vi "6517b+lakeshore335.vi"(8 "Set Temp Point":dbl=10.0, 11 "335 VISA resource name":refnum<visa-resource-name>="GPIB0::12::INSTR") -> ()   [LabVIEW 2019]
uses:
  lib/Lake Shore 335/Lake Shore 335.lvlib
  SubVI/SubVI.lvlib
  lib/Keithley 6517/Keithley 6517.lvlib
  <vilib>/Utility/file.llb/Write To Spreadsheet File (DBL).vi
  <vilib>/Utility/file.llb/Read From Spreadsheet File (DBL).vi
panel:
  out "Measurement":T1 {"Measurement" format="%.6e"}
  in  "VISA resource name":refnum<visa-resource-name>
  in  "采集最小间隔（ms）":u32
  in  "6157B":bool=TRUE
  out "Graph 2":cluster{"Y":dbl[], "Y":dbl[]}[](graph)
  out "Graph 1":cluster{"Y":dbl[], "Y":dbl[]}[](graph)
  in  "Y":u16(ring)=1 items=["时间", "通道A", "通道B", "电压", "电流", "电阻"]
  in  "X 2":u16(ring) items=["时间", "通道A", "通道B", "电压", "电流", "电阻"]
  in  "Y 2":u16(ring)=2 items=["时间", "通道A", "通道B", "电压", "电流", "电阻"]
  in  "X":u16(ring) items=["时间", "通道A", "通道B", "电压", "电流", "电阻"]
  out "Graph 3":cluster{"Y":dbl[], "Y":dbl[]}[](graph)
  out "Graph 4":cluster{"Y":dbl[], "Y":dbl[]}[](graph)
  in  "Y 3":u16(ring)=1 items=["时间", "通道A", "通道B", "电压", "电流", "电阻"]
  in  "X 3":u16(ring) items=["时间", "通道A", "通道B", "电压", "电流", "电阻"]
  in  "X 4":u16(ring) items=["时间", "通道A", "通道B", "电压", "电流", "电阻"]
  in  "Y 4":u16(ring)=2 items=["时间", "通道A", "通道B", "电压", "电流", "电阻"]
  in  "STOP":bool=TRUE
  out "date/time string":string="20171114204549"
  in  "file path (dialog if empty)":path
  in  "Range (0:Off)":u16(ring) items=["Off", "Low (On)", "Medium", "High"]
  in  "Heater Output (1:1)":u16(ring)=1 items=["1"=1, "2"=2]
  in  "Mode (0:Off)":u16(ring)=1 items=["Off", "Closed Loop PID", "Zone", "Open Loop", "Monitor Out", "Warmup Supply"]
  in  "Output Type (0:Current)":u16(ring) items=["Current", "Voltage"]
  in  "Power Up Enable (F: Off)":bool=TRUE
  in  "Input (0:None)":u16(ring)=2 items=["None", "A", "B"]
  in  "Max Current (0:User Specified)":u16(ring)=4 items=["User Specified", "0.707 A", "1.0 A", "1.141 A", "1.732 A"]
  in  "Max User Current (1.732)":dbl=1.0 format="%.3f"
  out "Heater Range":u16(ring) items=["Off", "Low (On)", "Medium", "High"]
  out "Heater Status":u16(ring) items=["No Error", "Heater Open Load", "Heater Short"]
  in  "Ramp Rate (0.0)":dbl=3.0 format="%.1f"
  in  "Enable Setpoint \nRamping (F: Off)":bool=TRUE
  # "K"
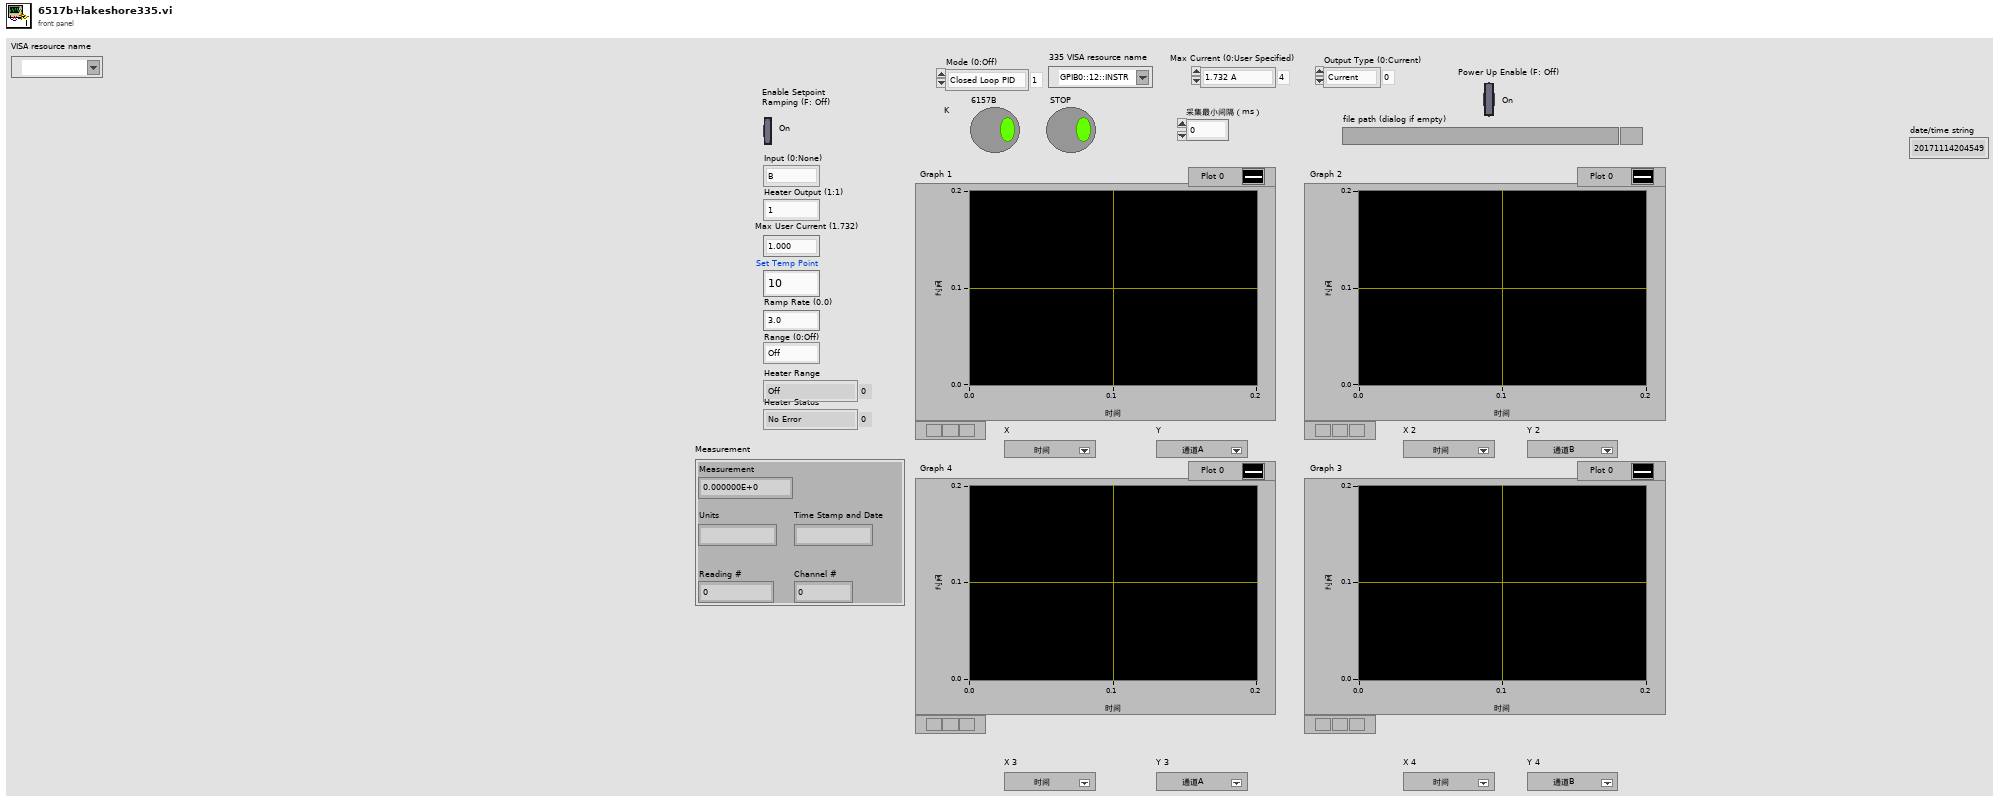
[diagram p1: front panel]
types:
  T1 = cluster{"Measurement":dbl, "Units":string, "Time Stamp and Date":string, "Reading #":dbl, "Channel #":dbl}
  T2 = enum16{"open", "replace", "create", "open or create", "replace or create", "replace or create with confirmation"}
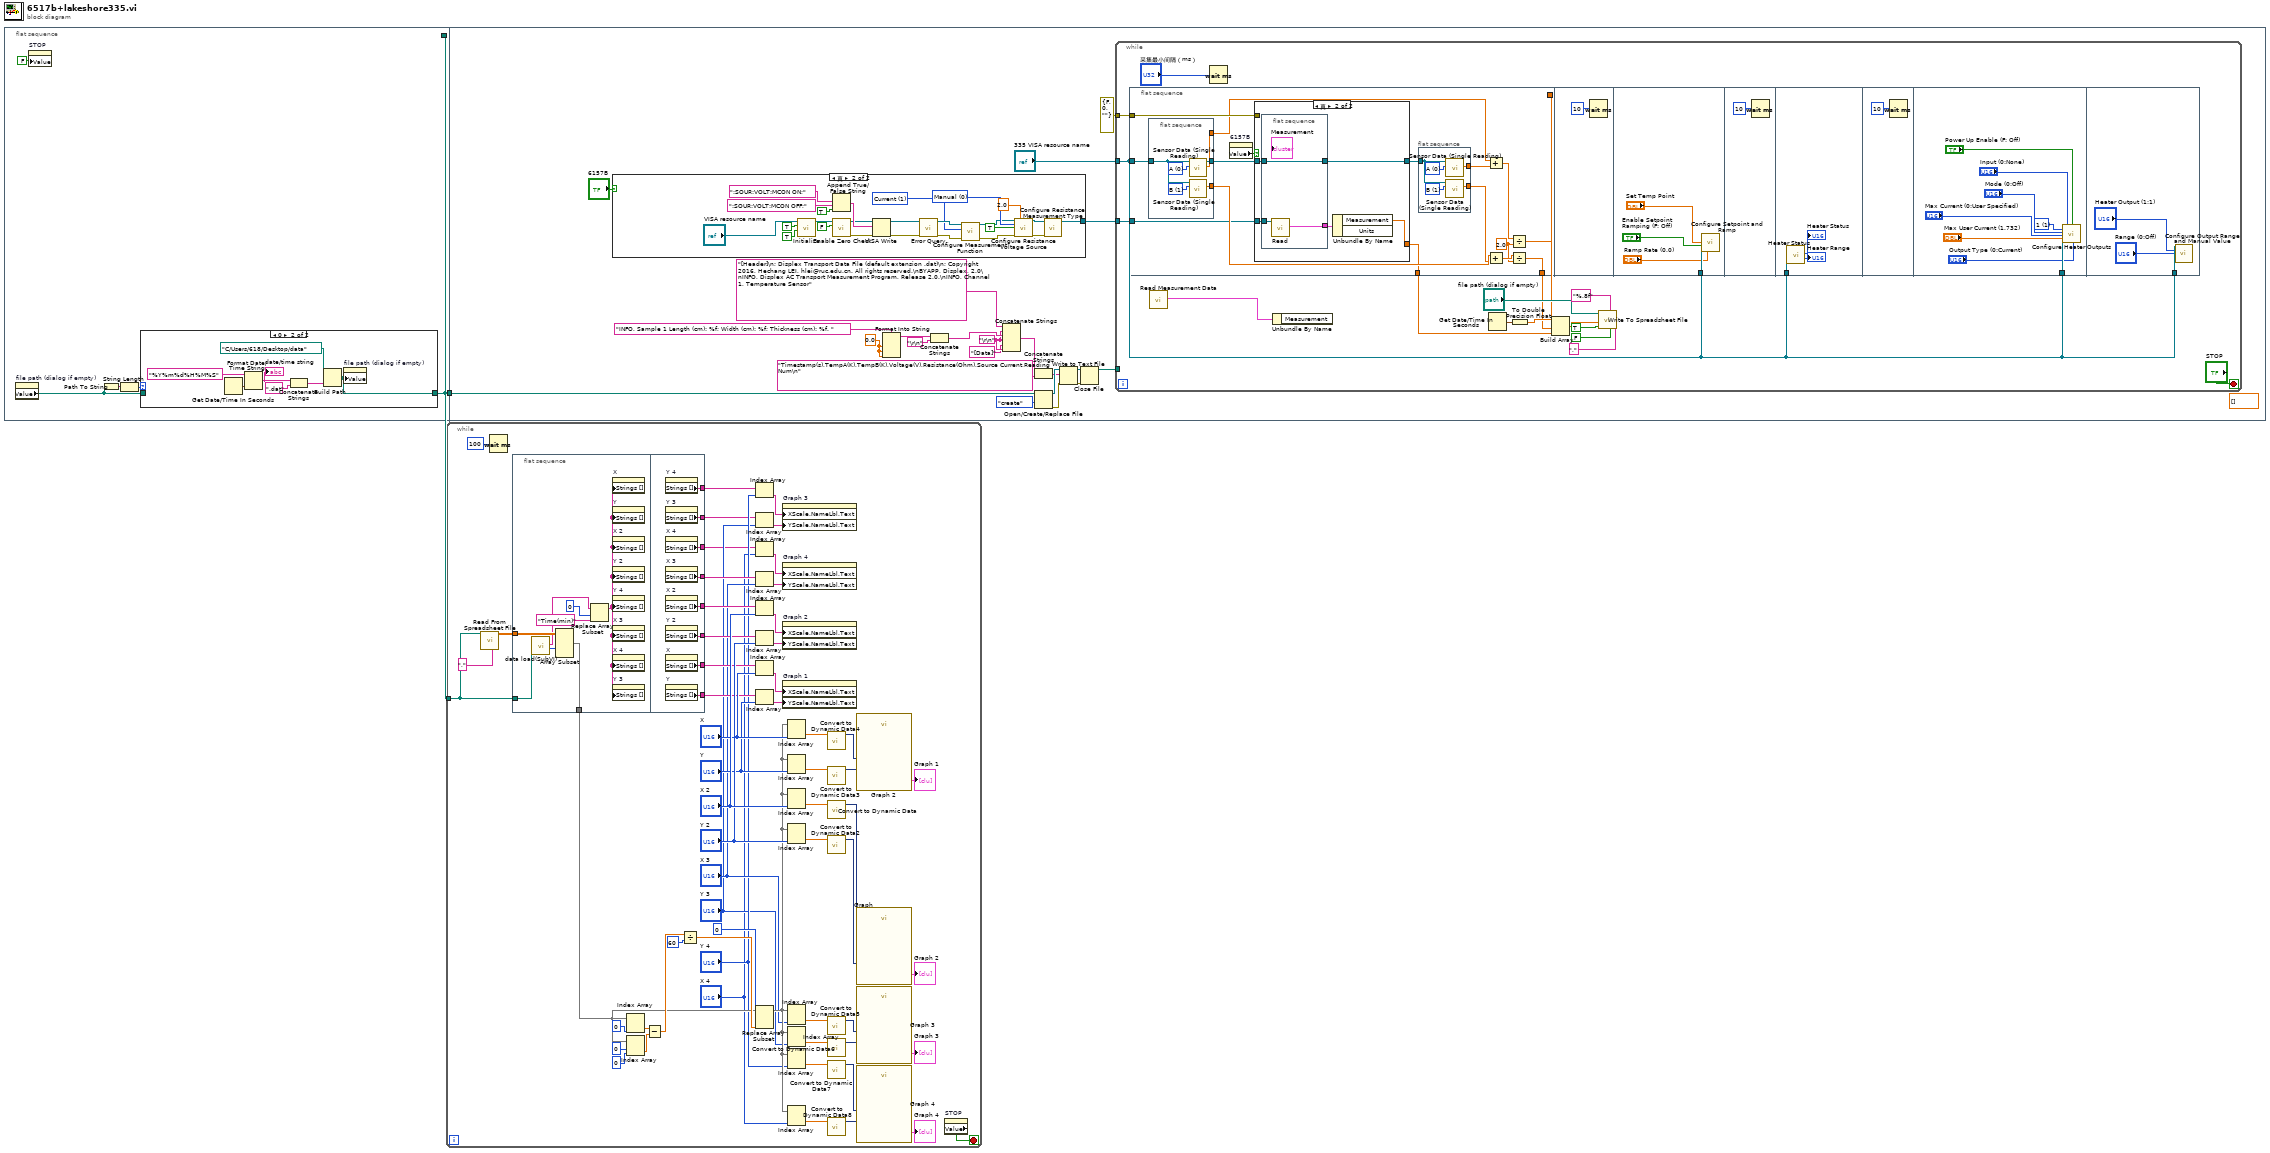
[diagram p0: block diagram]
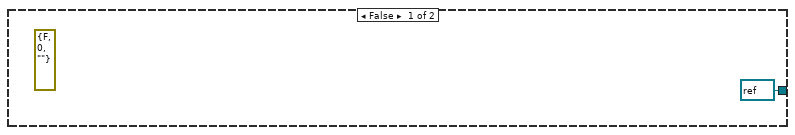
[diagram p3: hidden frame]
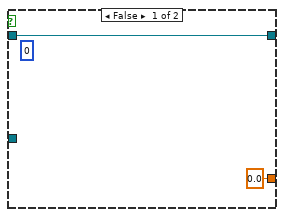
[diagram p4: hidden frame]
diagram:
  n1 = flat-sequence {
    tunnel: [w3] -> w1
    tunnel: [w3] -> w2
    tunnel: w2 -> [w35]
    frame #0 {
      n2 = property on="file path (dialog if empty)" class="Path"() -> ("Value"=w4:path)  [unwired: 2 in, 2 out]
      n3 = property on="STOP" class="Bool (严格)"("Value"=FALSE ("Boolean")) -> ()  [unwired: 2 in, 2 out]
      n4 = Path To String(path=w4) -> (string=w7:string)
      n5 = String Length(string=w7) -> (length=w6:i32)
      n6 = case shown="0" w6 {
        tunnel: [w8 w9] -> w3
        tunnel: w4 -> [w8 _]
        frame 1, Default {
        }
        frame 0 {
          n7 = Get Date/Time In Seconds() -> (seconds since 1Jan1904=w15:timestamp)
          n8 = Format Date/Time String(time format string (%c)="%Y%m%d%H%M%S", seconds (now)=w15) -> (date/time string=w10:string)  [unwired: 1 in]
          "date/time string" <- w10
          n9 = Concatenate Strings(w10, ".dat" ("string")) -> (w11:string)
          n10 = Build Path(base path=path "C:/Users/618/Desktop/data" ("文件夹路径"), name or relative path=w11) -> (appended path=w9:path)
          n11 = property on="file path (dialog if empty)" class="Path"("Value"=w9) -> ()  [unwired: 2 in, 2 out]
        }
      }
    }
    frame #1 {
      w24 = 0.0 ("输入 1")
      w27 = "\r\n"
      (unwired) dbl[] []
      n12 = case shown="真" "6157B" {
        tunnel: [refnum<visa-resource-name> refnum ("VISA resource name out") w39] -> w17
        frame False {
          (unwired) errorcluster {"status"=FALSE, "code"=0, "source"=""} ("error out")
        }
        frame True {
          w44 = 1 items=["Voltage", "Current", "Resistance", "Charge"] ("Measurement Function (0: Voltage)")
          w50 = 0 items=["Manual", "Auto"] ("Voltage Source Mode (0: Manual)")
          n13 = call "Initialize.vi"("Reset (True)"=TRUE, "ID Query (True)"=TRUE, "VISA resource name"="VISA resource name") -> ("VISA resource name out"=w42:refnum<visa-resource-name>)  [unwired: 7 in, 1 out]
          n14 = Append True/False String(1:TRUE ("Enable LO Connection (F: Disable)"), 2:":SOUR:VOLT:MCON OFF;", 3:":SOUR:VOLT:MCON ON;") -> (0:w59:string)  [unwired: 1 in]
          n15 = call "Enable Zero Check.vi"("Enable Zero Check (T: Enable)"=FALSE, "VISA resource name"=w42) -> ("error out"=w57:errorcluster, "VISA resource name out"=w58:refnum<visa-resource-name>)  [unwired: 8 in]
          n16 = VISA Write(VISA resource name=w58, write buffer=w59, error in (no error)=w57) -> (VISA resource name out=w56:refnum<visa-resource-name>, error out=w55:errorcluster)  [unwired: 1 out]
          n17 = call "Error Query.vi"("error in (no error)"=w55, "VISA resource name"=w56) -> ("error out"=w48:errorcluster, "VISA resource name out"=w47:refnum<visa-resource-name>)  [unwired: 6 in, 2 out]
          n18 = call "Configure Measurement Function.vi"("error in (no error)"=w48, "Measurement Function (0: Voltage)"=w44, "VISA resource name"=w47) -> ("error out"=w45:errorcluster, "VISA resource name out"=w46:refnum<visa-resource-name>)  [unwired: 7 in]
          n19 = call "Configure Resistance Voltage Source.vi"("VISA resource name"=w46, "Voltage Source Level (0.000000E+0)"=2.0, "Voltage Source Mode (0: Manual)"=w50, "Enable Voltage Source (F: Disable)"=TRUE, "error in (no error)"=w45) -> ("VISA resource name out"=w53:refnum<visa-resource-name>, "error out"=w52:errorcluster)  [unwired: 9 in]
          n20 = call "Configure Resistance Measurement Type.vi"("error in (no error)"=w52, "VISA resource name"=w53) -> ("VISA resource name out"=w39:refnum<visa-resource-name>)  [unwired: 8 in, 1 out]
        }
      }
      n21 = Format Into String(format string="INFO, Sample 1 Length (cm): %f; Width (cm): %f; Thickness (cm): %f. " ("string"), w24, w24, w24) -> (resulting string=w31:string)  [unwired: 2 in, 1 out]
      n22 = Concatenate Strings(w31, "\r\n") -> (w32:string)
      n23 = Concatenate Strings("[Header]\n; Displex Transport Data File (default extension .dat)\n; Copyright 2016, Hechang LEI, hlei@ruc.edu.cn. All rights reserved.\nBYAPP, Displex, 2.0\nINFO, Displex AC Transport Measurement Program, Release 2.0.\nINFO, Channel 1, Temperature Sensor" ("string"), w27, w32, w27, "[Data]" ("string"), w27) -> (w33:string)
      n24 = Concatenate Strings(w33, "Timestamp(s),TempA(K),TempB(K),Voltage(V),Resistance(Ohm),Source Current,Reading Num\n" ("字符串")) -> (w23:string)
      n25 = Open/Create/Replace File(file path (use dialog)=w35, operation (0:open)=T2."create") -> (refnum out=w34:refnum<file>, error out=w20:errorcluster)  [unwired: 4 in, 1 out]
      n26 = Write to Text File(file (use dialog)=w34, text=w23, error in=w20) -> (refnum out=w22:refnum<file>, error out=w21:errorcluster)  [unwired: 1 in, 1 out]
      n27 = Close File(refnum=w22, error in=w21) -> (path=w19:path)  [unwired: 1 out]
      n28 = while {
        tunnel: "335 VISA resource name" -> [w79]
        tunnel: w19 -> [_]
        tunnel: errorcluster {"status"=FALSE, "code"=0, "source"=""} ("error out") -> [w69]
        tunnel: w17 -> [w64]
        stop <- "STOP" stop-if-true
        n29 = flat-sequence {
          tunnel: w79 -> [w95]
          tunnel: w69 -> [w94]
          tunnel: [w84] -> w68
          tunnel: [w83] -> w67
          tunnel: [w82] -> w66
          tunnel: w64 -> [w80]
          tunnel: w79 -> [w121]
          tunnel: w79 -> [w125]
          tunnel: w79 -> [w134]
          tunnel: w79 -> [w137]
          frame #0 {
            w88 = 2.0 ("y")
            n30 = flat-sequence {
              tunnel: w95 -> [w109]
              tunnel: [w108] -> w87
              tunnel: [w107] -> w91
              tunnel: [w106] -> w85
              frame #0 {
                w110 = u16 1 items=["A", "B"] ("Input (0:A)")
                w111 = u16 0 items=["A", "B"] ("Input (0:A)")
                n31 = call "Sensor Data (Single Reading).vi"("Input (0:A)"=w111, "VISA resource name"=w109) -> ("Sensor Data"=w108:dbl, "VISA resource name out"=w106:refnum<visa-resource-name>)  [unwired: 7 in, 1 out]
                n32 = call "Sensor Data (Single Reading).vi"("Input (0:A)"=w110, "VISA resource name"=w109) -> ("Sensor Data"=w107:dbl)  [unwired: 7 in, 2 out]
              }
            }
            n33 = property on="6157B" class="Bool (严格)"() -> ("Value"=w81:bool)  [unwired: 2 in, 2 out]
            n34 = case shown="真" w81 {
              tunnel: w94 -> [_ _]
              tunnel: [w96 w100] -> w93
              tunnel: w85 -> [w96 w101]
              tunnel: [sgl 0.0 w102] -> w82
              tunnel: w80 -> [_ w99]
              frame False {
                (unwired) u32 0
              }
              frame True {
                n35 = flat-sequence {
                  tunnel: w101 -> [w105]
                  tunnel: [w105] -> w100
                  tunnel: w99 -> [w104]
                  tunnel: [w103] -> w98
                  frame #0 {
                    n36 = call "Read.vi"("VISA resource name"=w104) -> ("Measurement"=w103:T1)  [unwired: 8 in, 2 out]
                  }
                }
                n37 = Unbundle By Name(w98) -> ("Measurement"=w102:dbl)  [unwired: 1 out]
              }
            }
            n38 = flat-sequence {
              tunnel: w93 -> [w114]
              tunnel: [w113] -> w90
              tunnel: [w112] -> w86
              frame #0 {
                w116 = u16 1 items=["A", "B"] ("Input (0:A)")
                w115 = u16 0 items=["A", "B"] ("Input (0:A)")
                n39 = call "Sensor Data (Single Reading).vi"("Input (0:A)"=w115, "VISA resource name"=w114) -> ("Sensor Data"=w112:dbl)  [unwired: 7 in, 2 out]
                n40 = call "Sensor Data (Single Reading).vi"("Input (0:A)"=w116, "VISA resource name"=w114) -> ("Sensor Data"=w113:dbl)  [unwired: 7 in, 2 out]
              }
            }
            n41 = Add(x=w87, y=w86) -> (x+y=w89:dbl)
            n42 = Add(x=w91, y=w90) -> (x+y=w92:dbl)
            n43 = Divide(x=w89, y=w88) -> (x/y=w84:dbl)
            n44 = Divide(x=w92, y=w88) -> (x/y=w83:dbl)
          }
          frame #1 {
            n45 = Wait (ms)(milliseconds to wait=u32 10 ("等待时间（毫秒）")) -> ()  [unwired: 1 out]
          }
          frame #2 {
            n46 = call "Configure Setpoint and Ramp.vi"("VISA resource name"=w121, "Setpoint (0.0000)"="Set Temp Point", "Enable Setpoint Ramping (F: Off)"="Enable Setpoint \nRamping (F: Off)", "Ramp Rate (0.0)"="Ramp Rate (0.0)") -> ()  [unwired: 10 in, 2 out]
          }
          frame #3 {
            n47 = Wait (ms)(milliseconds to wait=u32 10 ("等待时间（毫秒）")) -> ()  [unwired: 1 out]
          }
          frame #4 {
            n48 = call "Heater Status.vi"("VISA resource name"=w125) -> ("Heater Range"=→"Heater Range":u16, "Heater Status"=→"Heater Status":u16)  [unwired: 6 in, 3 out]
          }
          frame #5 {
            n49 = Wait (ms)(milliseconds to wait=u32 10 ("等待时间（毫秒）")) -> ()  [unwired: 1 out]
          }
          frame #6 {
            w133 = u16 1 items=["1"=1, "2"=2] ("Heater Output (1:1)")
            n50 = call "Configure Heater Outputs.vi"("VISA resource name"=w134, "Heater Output (1:1)"=w133, "Mode (0:Off)"="Mode (0:Off)", "Max Current (0:User Specified)"="Max Current (0:User Specified)", "Max User Current (1.732)"="Max User Current (1.732)", "Input (0:None)"="Input (0:None)", "Power Up Enable (F: Off)"="Power Up Enable (F: Off)", "Output Type (0:Current)"="Output Type (0:Current)") -> ()  [unwired: 10 in, 2 out]
          }
          frame #7 {
            n51 = call "Configure Output Range and Manual Value.vi"("VISA resource name"=w137, "Heater Output (1:1)"="Heater Output (1:1)", "Range (0:Off)"="Range (0:Off)") -> ()  [unwired: 11 in, 2 out]
          }
        }
        n52 = call "Read Measurement Data.vi"() -> ("Measurement"=w63:T1)  [unwired: 9 in, 2 out]
        n53 = Wait (ms)(milliseconds to wait="采集最小间隔（ms）") -> ()  [unwired: 1 out]
        n54 = Unbundle By Name(w63) -> ()  [unwired: 1 out]
        n55 = Get Date/Time In Seconds() -> (seconds since 1Jan1904=w72:timestamp)
        n56 = To Double Precision Float(number=w72) -> (double precision float=w71:dbl)
        n57 = Build Array(w71, w68, w67, w66) -> (w74:dbl[])
        n58 = call-poly <vilib>:"Write To Spreadsheet File.vi"("delimiter (\\t)"="," ("delimiter (\\t)"), "transpose? (no:F)"=FALSE, "format (%.3f)"="%.8f", "append to file? (new file:F)"=TRUE, "1D data"=w74, "file path (dialog if empty)"="file path (dialog if empty)") -> ()  [unwired: 2 in, 1 out]
      }
    }
  }
  n59 = while {
    tunnel: w1 -> [w151]
    stop <- w138 stop-if-true
    n60 = call-poly <vilib>:"Read From Spreadsheet File.vi"("delimiter (\\t)"="," ("delimiter (\\t)"), "file path (dialog if empty)"=w151) -> ("all rows"=w164:dbl[][])  [unwired: 5 in, 4 out]
    n61 = Wait (ms)(milliseconds to wait=u32 100) -> ()  [unwired: 1 out]
    n62 = flat-sequence {
      tunnel: w151 -> [w204]
      tunnel: w164 -> [w203]
      tunnel: [w202] -> w163
      tunnel: [w213] -> w168
      tunnel: [w212] -> w167
      tunnel: [w211] -> w166
      tunnel: [w210] -> w165
      tunnel: [w209] -> w150
      tunnel: [w208] -> w148
      tunnel: [w207] -> w146
      tunnel: [w206] -> w142
      frame #0 {
        n63 = call "data load(SubVI).vi"("file path"=w204) -> ("数据起始行"=w205:i32, "项名"=w201:string[])  [unwired: 9 in]
        n64 = Array Subset(array=w203, index (row)=w205) -> (w202:dbl[][])  [unwired: 3 in]
        n65 = Replace Array Subset(array=w201, new element="Time(min)" ("new element/subarray"), index=0) -> (w198:string[])
        n66 = property on="X" class="Ring (严格)"("Strings []"=w198) -> ()  [unwired: 2 in, 2 out]
        n67 = property on="Y" class="Ring (严格)"("Strings []"=w198) -> ()  [unwired: 2 in, 2 out]
        n68 = property on="X 2" class="Ring (严格)"("Strings []"=w198) -> ()  [unwired: 2 in, 2 out]
        n69 = property on="Y 2" class="Ring (严格)"("Strings []"=w198) -> ()  [unwired: 2 in, 2 out]
        n70 = property on="Y 4" class="Ring (严格)"("Strings []"=w198) -> ()  [unwired: 2 in, 2 out]
        n71 = property on="X 3" class="Ring (严格)"("Strings []"=w198) -> ()  [unwired: 2 in, 2 out]
        n72 = property on="X 4" class="Ring (严格)"("Strings []"=w198) -> ()  [unwired: 2 in, 2 out]
        n73 = property on="Y 3" class="Ring (严格)"("Strings []"=w198) -> ()  [unwired: 2 in, 2 out]
      }
      frame #1 {
        n74 = property on="Y 4" class="Ring (严格)"() -> ("Strings []"=w208:string[])  [unwired: 2 in, 2 out]
        n75 = property on="Y 3" class="Ring (严格)"() -> ("Strings []"=w207:string[])  [unwired: 2 in, 2 out]
        n76 = property on="X 4" class="Ring (严格)"() -> ("Strings []"=w206:string[])  [unwired: 2 in, 2 out]
        n77 = property on="X 3" class="Ring (严格)"() -> ("Strings []"=w209:string[])  [unwired: 2 in, 2 out]
        n78 = property on="X 2" class="Ring (严格)"() -> ("Strings []"=w212:string[])  [unwired: 2 in, 2 out]
        n79 = property on="Y 2" class="Ring (严格)"() -> ("Strings []"=w210:string[])  [unwired: 2 in, 2 out]
        n80 = property on="X" class="Ring (严格)"() -> ("Strings []"=w213:string[])  [unwired: 2 in, 2 out]
        n81 = property on="Y" class="Ring (严格)"() -> ("Strings []"=w211:string[])  [unwired: 2 in, 2 out]
      }
    }
    n82 = Index Array(array=w163, index (col)=0 ("disabled index (col)")) -> (element=w177:dbl[])  [unwired: 1 in]
    n83 = Index Array(array=w163, index (row)=0 ("disabled index (row)"), index (col)=0 ("disabled index (col)")) -> (element=w178:dbl)
    n84 = Subtract(x=w177, y=w178) -> (x-y=w171:dbl[])
    n85 = Divide(x=w171, y=60) -> (x/y=w170:dbl[])
    n86 = Index Array(array=w148, index="Y 4") -> (element=w144:string)
    n87 = Index Array(array=w146, index="Y 3") -> (element=w143:string)
    n88 = Index Array(array=w142, index="X 4") -> (element=w140:string)
    n89 = Index Array(array=w150, index="X 3") -> (element=w139:string)
    n90 = Index Array(array=w167, index="X 2") -> (element=w188:string)
    n91 = Index Array(array=w165, index="Y 2") -> (element=w187:string)
    n92 = Index Array(array=w168, index="X") -> (element=w190:string)
    n93 = Index Array(array=w166, index="Y") -> (element=w189:string)
    n94 = Replace Array Subset(array=w163, new element=w170, index (col)=0 ("disabled index (col)")) -> (w160:dbl[][])  [unwired: 1 in]
    n95 = property on="Graph 3" class="XYGraph (严格)"("XScale.NameLbl.Text"=w144, "YScale.NameLbl.Text"=w143) -> ()  [unwired: 2 in, 2 out]
    n96 = property on="Graph 4" class="XYGraph (严格)"("XScale.NameLbl.Text"=w140, "YScale.NameLbl.Text"=w139) -> ()  [unwired: 2 in, 2 out]
    n97 = property on="Graph 2" class="XYGraph (严格)"("XScale.NameLbl.Text"=w188, "YScale.NameLbl.Text"=w187) -> ()  [unwired: 2 in, 2 out]
    n98 = property on="Graph 1" class="XYGraph (严格)"("XScale.NameLbl.Text"=w190, "YScale.NameLbl.Text"=w189) -> ()  [unwired: 2 in, 2 out]
    n99 = Index Array(array=w160, index (col)="X") -> (element=w175:dbl[])  [unwired: 1 in]
    n100 = Index Array(array=w160, index (col)="Y") -> (element=w192:dbl[])  [unwired: 1 in]
    n101 = Index Array(array=w160, index (col)="X 2") -> (element=w185:dbl[])  [unwired: 1 in]
    n102 = Index Array(array=w160, index (col)="Y 2") -> (element=w194:dbl[])  [unwired: 1 in]
    n103 = Index Array(array=w160, index (col)="X 3") -> (element=w159:dbl[])  [unwired: 1 in]
    n104 = Index Array(array=w160, index (col)="Y 3") -> (element=w157:dbl[])  [unwired: 1 in]
    n105 = Index Array(array=w160, index (col)="Y 4") -> (element=w155:dbl[])  [unwired: 1 in]
    n106 = Index Array(array=w160, index (col)="X 4") -> (element=w153:dbl[])  [unwired: 1 in]
    n107 = call "Convert to Dynamic Data4"("Array"=w175) -> ("Dynamic Data Type"=w174:dynamicdata)  [unwired: 3 in]
    n108 = call "Convert to Dynamic Data3"("Array"=w192) -> ("Dynamic Data Type"=w191:dynamicdata)  [unwired: 3 in]
    n109 = call "Convert to Dynamic Data"("Array"=w185) -> ("Dynamic Data Type"=w195:dynamicdata)  [unwired: 3 in]
    n110 = call "Convert to Dynamic Data2"("Array"=w194) -> ("Dynamic Data Type"=w193:dynamicdata)  [unwired: 3 in]
    n111 = call "Convert to Dynamic Data5"("Array"=w159) -> ("Dynamic Data Type"=w158:dynamicdata)  [unwired: 3 in]
    n112 = call "Convert to Dynamic Data6"("Array"=w157) -> ("Dynamic Data Type"=w156:dynamicdata)  [unwired: 3 in]
    n113 = call "Convert to Dynamic Data7"("Array"=w155) -> ("Dynamic Data Type"=w154:dynamicdata)  [unwired: 3 in]
    n114 = call "Convert to Dynamic Data8"("Array"=w153) -> ("Dynamic Data Type"=w152:dynamicdata)  [unwired: 3 in]
    n115 = call "Graph 2"("Y Input"=w191, "X Input"=w174) -> ("XY Graph"=→"Graph 1":cluster{"Y":dbl[], "Y":dbl[]}[])  [unwired: 3 in, 6 out]
    n116 = call "Graph"("Y Input"=w193, "X Input"=w195) -> ("XY Graph"=→"Graph 2":cluster{"Y":dbl[], "Y":dbl[]}[])  [unwired: 3 in, 6 out]
    n117 = call "Graph 3"("Y Input"=w156, "X Input"=w158) -> ("XY Graph"=→"Graph 3":cluster{"Y":dbl[], "Y":dbl[]}[])  [unwired: 3 in, 6 out]
    n118 = call "Graph 4"("Y Input"=w152, "X Input"=w154) -> ("XY Graph"=→"Graph 4":cluster{"Y":dbl[], "Y":dbl[]}[])  [unwired: 3 in, 6 out]
    n119 = property on="STOP" class="Bool (严格)"() -> ("Value"=w138:bool)  [unwired: 2 in, 2 out]
  }
